vi "difftool config key.vi"() -> (3 "difftool key":string)   [LabVIEW 2016]
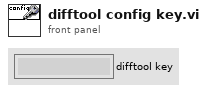
[diagram p1: front panel]
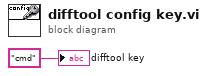
[diagram p0: block diagram]
diagram:
  "difftool key" <- "cmd"
